vi "Destroy Multiplexed Messenger.vi"(8 "error in (no error)":errorcluster, 11 "Multiplexed Messenger In":refnum<data-value>) -> (0 "error out":errorcluster)   [LabVIEW 2019, in "Network Messenger.lvlib" / "Multiplexed Messenger.lvclass"]
uses:
  <vilib>/gpm_packages/@cs/Network-interface/Source/Network Messenger/Multiplexed Messenger/Multiplexed Messenger.lvclass
  <vilib>/gpm_packages/@cs/Network-interface/Source/Network Messenger/Multiplexed Messenger/Multiplexed Messenger.lvclass/Multiplexed Messenger.ctl
  <vilib>/ActorFramework/Message Enqueuer/Message Enqueuer.lvclass/Message Enqueuer.ctl
  <vilib>/ActorFramework/Message Enqueuer/Enqueue.vi
  <vilib>/ActorFramework/Stop Msg/Stop Msg.lvclass
  C:/Program Files/National Instruments/LabVIEW 2019/vi.lib/ActorFramework/Message/Message.lvclass
  <vilib>/ActorFramework/Message Priority Queue/Priority Enqueue.vi
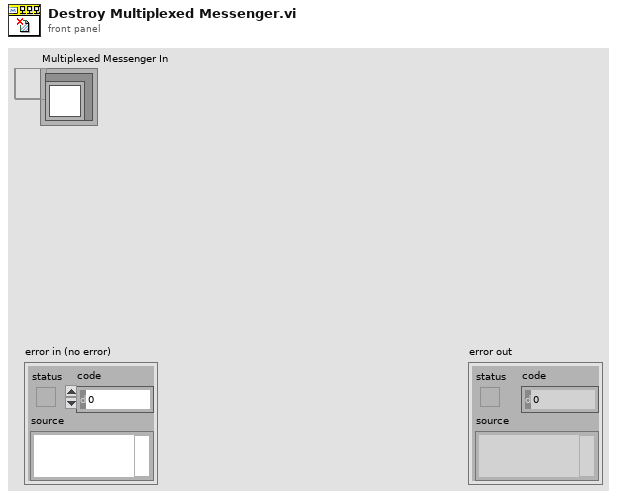
[diagram p1: front panel]
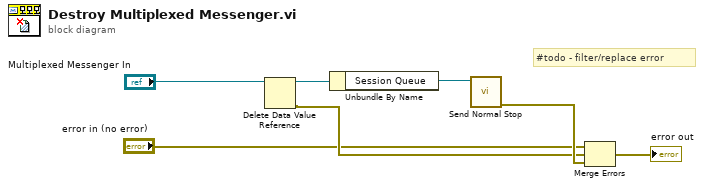
[diagram p0: block diagram]
diagram:
  # "#todo - filter/replace error"
  n1 = Delete Data Value Reference(data value reference="Multiplexed Messenger In") -> (data value=w4:refnum<class "Multiplexed Messenger.lvclass">, error out=w3:errorcluster)  [unwired: 1 in]
  n2 = Unbundle By Name(w4) -> ("Session Queue"=w6:refnum<class "Message Enqueuer.lvclass">)
  n3 = call <vilib>:"Send Normal Stop.vi"("Message Enqueuer"=w6) -> ("error out"=w5:errorcluster)  [unwired: 10 in]
  n4 = Merge Errors("error in (no error)", w3, w5) -> (→"error out":errorcluster)
